vi "Get_Config_Data.vi"(8 "error in (no error)":errorcluster, 11 "USB-87Pn_Data In":T1) -> (0 "error out":errorcluster, 3 "USB-87Pn_Data Out":T1)   [LabVIEW 2019, in "USB-87P8_Manager.lvlib"]
uses:
  USB-87P8_Manager.lvlib
  Actor/USB-87Pn_Data.ctl
  USB-87Pn.lvclass
  <vilib>/Utility/config.llb/Read Key (I32).vi
  <vilib>/Utility/config.llb/NI_LVConfig.lvlib
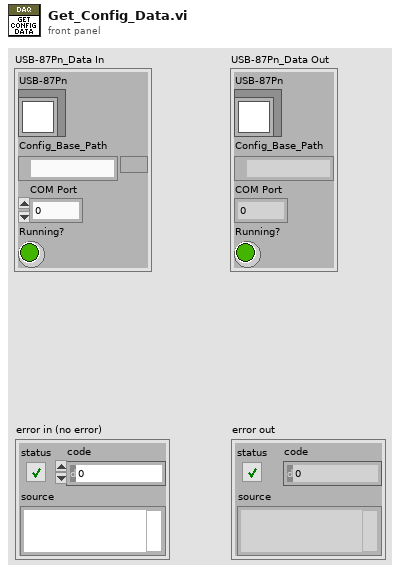
[diagram p1: front panel]
types:
  T1 = typedef "USB-87P8_Manager.lvlib/USB-87Pn_Data.ctl" = cluster{"USB-87Pn":refnum<class "USB-87Pn.lvclass">, "Config_Base_Path":path, "COM Port":i32, "Running?":bool}
  T2 = typedef "NI_LVConfig.lvlib/Config Data RefNum.ctl" = refnum<k1>
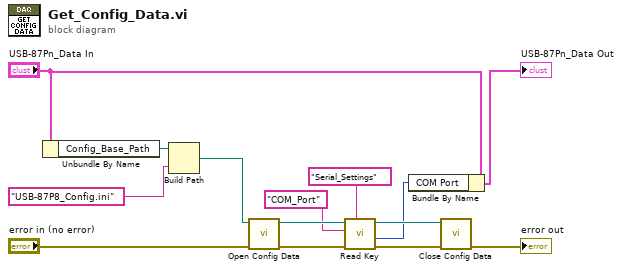
[diagram p0: block diagram]
diagram:
  n1 = Unbundle By Name("USB-87Pn_Data In") -> ("Config_Base_Path"=w13:path)
  n2 = Build Path(base path=w13, name or relative path="USB-87P8_Config.ini") -> (appended path=w12:path)
  n3 = call <vilib>:"Open Config Data.vi"("error in (no error)"="error in (no error)", "configuration file path"=w12) -> ("error out"=w9:errorcluster, "refnum"=w10:T2)  [unwired: 7 in, 1 out]
  n4 = call-poly <vilib>:"Read Key.vi"("section"="Serial_Settings", "error in (no error)"=w9, "key"="COM_Port", "refnum"=w10) -> ("error out"=w7:errorcluster, "value"=w2:i32, "refnum out"=w8:T2)  [unwired: 4 in, 1 out]
  n5 = Bundle By Name(cluster="USB-87Pn_Data In", "COM Port"=w2) -> (→"USB-87Pn_Data Out":T1)
  n6 = call <vilib>:"Close Config Data.vi"("error in (no error)"=w7, "refnum"=w8) -> ("error out"=→"error out":errorcluster)  [unwired: 8 in, 1 out]
